vi "Log Waveform Data.vi"(0 "Data Logger Interface in":refnum<class "TDMS Data Logger Actor.lvclass">, 5 "Group Name (Untitled)":string, 7 "Channel Names (Untitled)":string[](array[string]), 9 "Data":waveform(dbl)[](array[waveform]), 11 "error in (no error)":errorcluster) -> (4 "Data Logger Interface out":refnum<class "TDMS Data Logger Actor.lvclass">, 15 "error out":errorcluster)   [LabVIEW 2024, in "TDMS Data Logger Actor.lvlib" / "TDMS Data Logger Actor.lvclass"]
uses:
  TDMS Data Logger Actor.lvclass
  TDMS Data Logger Actor.lvclass/TDMS Data Logger Actor.ctl
  Logging Data/1D Waveform Logging Data/1D Waveform Logging Data.lvclass
  C:/Users/uspoaotto/OneDrive - Oregon Tool/Desktop/working copies/dataLogger/Logging Data Interface/Logging Data Interface/Logging Data Interface.lvclass
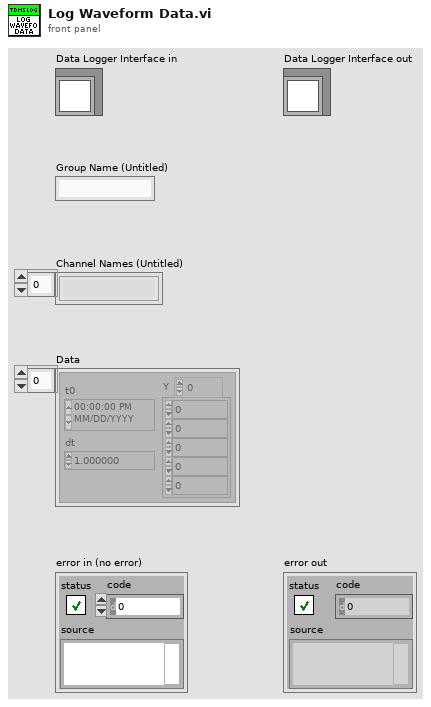
[diagram p1: front panel]
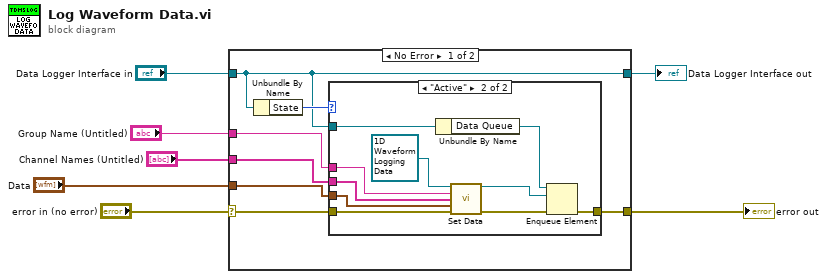
[diagram p0: block diagram]
diagram:
  n1 = case shown="No Error" "error in (no error)" {
    selector: "error in (no error)" -> [w11 w26]
    tunnel: "Data Logger Interface in" -> [w13 w27]
    tunnel: "Channel Names (Untitled)" -> [w9 _]
    tunnel: "Group Name (Untitled)" -> [w10 _]
    tunnel: "Data" -> [w8 _]
    tunnel: [w13 w27] -> w2
    tunnel: [w12 w26] -> w1
    frame No Error {
      n2 = Unbundle By Name(w13) -> ("State"=w14:enum16{"Idle", "Active", "Paused"})
      n3 = case shown="\"Active\"" w14 {
        tunnel: w13 -> [_ w25]
        tunnel: [w15 w23] -> w12
        tunnel: w11 -> [w15 w18]
        tunnel: w10 -> [_ w21]
        tunnel: w9 -> [_ w20]
        tunnel: w8 -> [_ w19]
        frame "Idle", "Paused" {
        }
        frame "Active" {
          n4 = Unbundle By Name(w25) -> ("Data Queue"=w24:refnum<queue>)
          n5 = call "Set Data.vi"("1D Waveform Data in"=refnum<class "1D Waveform Logging Data.lvclass"> refnum, "Group Name"=w21, "Channel Names"=w20, "Data"=w19, "error in (no error)"=w18) -> ("1D Waveform Data out"=w16:refnum<class "1D Waveform Logging Data.lvclass">, "error out"=w17:errorcluster)  [unwired: 9 in]
          n6 = Enqueue Element(queue=w24, element=w16, error in (no error)=w17) -> (error out=w23:errorcluster)  [unwired: 1 in, 2 out]
        }
      }
    }
    frame Error {
    }
  }
  "error out" <- w1
  "Data Logger Interface out" <- w2
